vi "Servo SSC.vi"(0 "VISA resource name":refnum<visa-resource-name>="COM1", 6 "Read":bool) -> ()   [LabVIEW 2011]
doc: "The Basic Serial Read and Write example performs a Serial Port Read, a Serial Port Write, or a combination of these actions. The user selects the actions (read or write) on the front panel. If both are selected, the VI will write the data first, read data, and then close the VISA session that is opened to the port. This VI will wait until the specified number of bytes is received at the port. Only the number of bytes specified will be read.\n\nINSTRUCTIONS:\n1) Select the serial resource and configuration parameters (baud rate, data bits, parity, stop bits, flow control).\n2) Select the operations to be performed. \n3) Connect the serial port to your device. If no device is available, perform a loopback test by doing one of the following. Short pins 2 and 3 on a RS-232 cable or short pin 4 to pin 8 and pin 5 to pin 9 on a RS-485/422 cable. \n4) Run the VI to see the data read. (The \"read string\" will match the \"string to write\" if a loopback test was performed.)\n\nNote: The parameters set for the serial port must match the parameters of the connected instrument or device. In this example, the bytes to read parameter specifies the number of bytes that the serial port reads. If there were more bytes at the port than the number specified in bytes to read, those bytes would not be read. Also, if you specify to read more bytes than the number of bytes actually read, you might receive a timeout error message.\n\nOn the block diagram, the Configure Serial Port VI sets the configuration parameters. The front panel displays the controls used to configure the basic parameters, such as baud rate, data bits, and parity. Constants configure the other parameters the user probably does not need set. After the VISA Configure Serial Port VI opens the VISA session and configures the port, the VI passes the VISA resource name to other VIs that perform operations on that VISA resource. The VISA Write function sends a command to the serial device and the VISA Read function returns data based on the command. The VISA Close function then closes the reference to the serial device. It is important to close the reference; otherwise communication through with that port through protocols other than VISA might not be possible."
uses:
  <vilib>/Instr/_visa.llb/VISA Configure Serial Port (Instr).vi
panel:
  out "value 2":u8
  in  "delay before read (ms)":u32=25
  in  "string to write":string="va \n"
  out "bytes read":u32
  out "read string":string
  out "value 1":u8
  out "Waveform Chart":T1(graph)
  in  "SERVO 4":dbl(knob)=1500.0 scale=500.0..2500.0
  in  "SERVO 3":dbl(knob)=1500.0 scale=500.0..2500.0
  in  "SERVO 2":dbl(knob)=1500.0 scale=500.0..2500.0
  in  "SERVO 1":dbl(knob)=1500.0 scale=500.0..2500.0
  in  "SERVO 0":dbl(knob)=1500.0 scale=500.0..2500.0
  in  "Initial":bool
  in  "Time":dbl=500.0
  in  "Write":bool
  out "Result":string
  in  "stop":bool
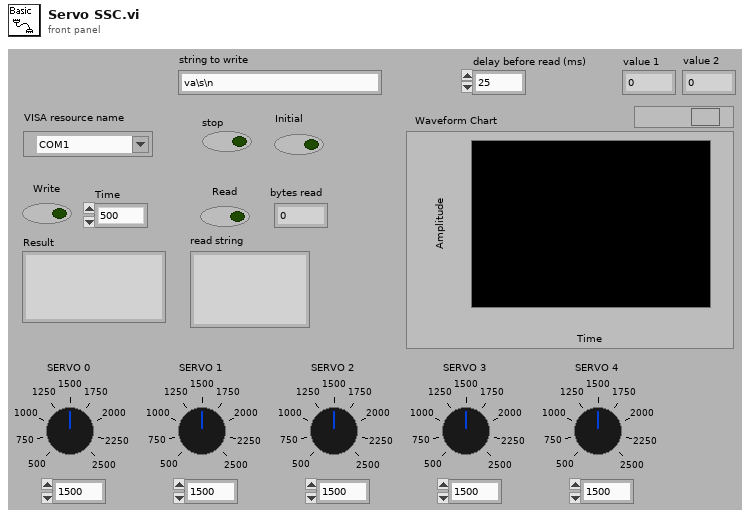
[diagram p1: front panel]
types:
  T1 = cluster{"unsigned byte array[0]":u8, "unsigned byte array[1]":u8, "unsigned byte array[2]":u8, "unsigned byte array[3]":u8, "unsigned byte array[4]":u8, "unsigned byte array[5]":u8, "unsigned byte array[6]":u8, "unsigned byte array[7]":u8, "unsigned byte array[8]":u8, "unsigned byte array[9]":u8, "unsigned byte array[10]":u8, "unsigned byte array[11]":u8, "unsigned byte array[12]":u8, "unsigned byte array[13]":u8, "unsigned byte array[14]":u8, "unsigned byte array[15]":u8, "unsigned byte array[16]":u8, "unsigned byte array[17]":u8}
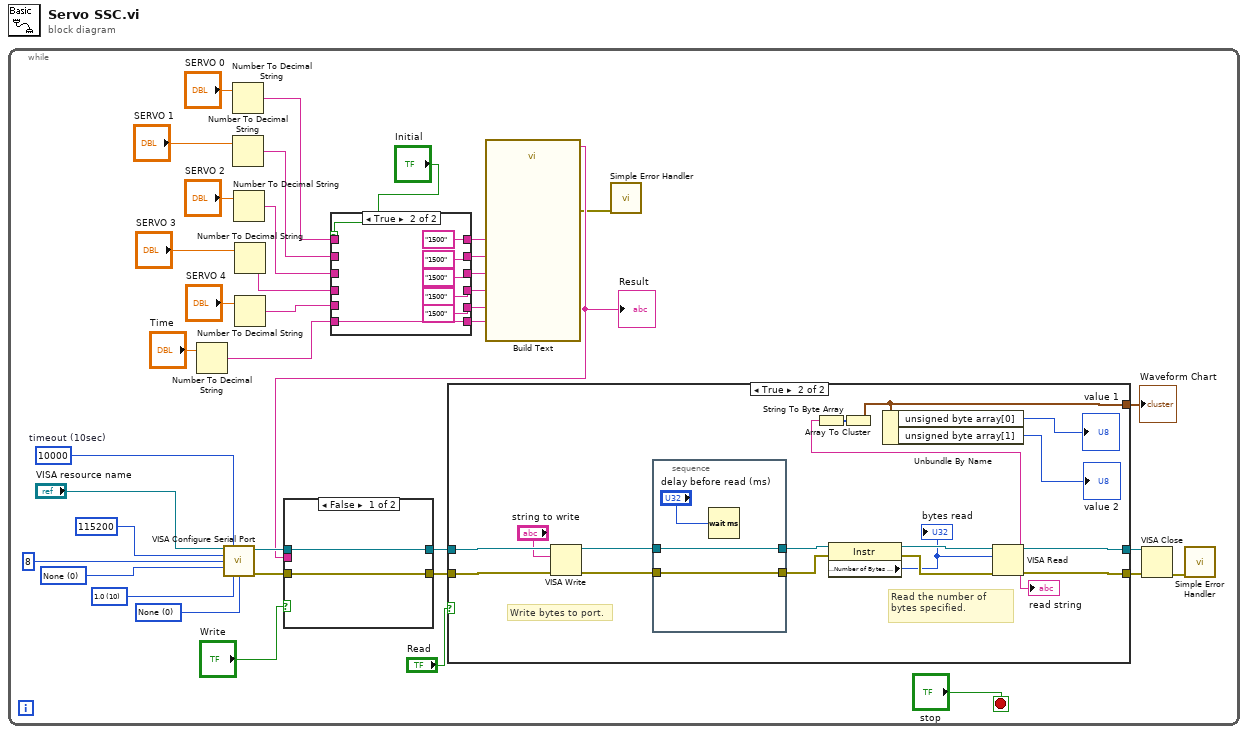
[diagram p0: block diagram]
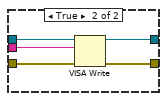
[diagram p3: hidden frame]
diagram:
  n1 = while {
    stop <- "stop" stop-if-true
    w33 = u16 0 items=["None"=0, "XON/XOFF"=1, "RTS/CTS"=2, "DTR/DSR"=4] ("flow control")
    w34 = u16 10 items=["1.0"=10, "1.5"=15, "2.0"=20] ("stop bits")
    w36 = u16 0 items=["None", "Odd", "Even", "Mark", "Space"] ("parity")
    w35 = u32 10000  # timeout (10sec)
    n2 = Number To Decimal String(number="Time") -> (decimal integer string=w21:string)  [unwired: 1 in]
    n3 = call-poly "VISA Configure Serial Port"("VISA resource name"="VISA resource name", "timeout (10sec)"=w35, "baud rate (9600)"=u32 115200 ("baud rate"), "data bits (8)"=u16 8 ("data bits"), "parity (0:none)"=w36, "stop bits (10: 1 bit)"=w34, "flow control (0:none)"=w33) -> ("VISA resource name out"=w31:refnum<visa-resource-name>, "error out"=w30:errorcluster)  [unwired: 7 in]
    n4 = Number To Decimal String(number="SERVO 0") -> (decimal integer string=w18:string)  [unwired: 1 in]
    n5 = Number To Decimal String(number="SERVO 1") -> (decimal integer string=w19:string)  [unwired: 1 in]
    n6 = Number To Decimal String(number="SERVO 2") -> (decimal integer string=w20:string)  [unwired: 1 in]
    n7 = Number To Decimal String(number="SERVO 3") -> (decimal integer string=w23:string)  [unwired: 1 in]
    n8 = Number To Decimal String(number="SERVO 4") -> (decimal integer string=w22:string)  [unwired: 1 in]
    n9 = case shown="True" "Initial" {
      tunnel: w23 -> [w43 _]
      tunnel: w22 -> [w44 _]
      tunnel: w21 -> [w45 w51]
      tunnel: w20 -> [w42 _]
      tunnel: w19 -> [w41 _]
      tunnel: w18 -> [w40 _]
      tunnel: [w45 w51] -> w17
      tunnel: [w44 "1500"] -> w16
      tunnel: [w43 "1500"] -> w15
      tunnel: [w42 "1500"] -> w14
      tunnel: [w41 "1500"] -> w13
      tunnel: [w40 "1500"] -> w12
      frame False {
      }
      frame True {
      }
    }
    n10 = call "Build Text"("pwm3"=w15, "time"=w17, "pwm0"=w12, "pwm1"=w13, "pwm2"=w14, "pwm4"=w16) -> ("Result"=w25:string, "error out"=w11:errorcluster)  [unwired: 8 in]
    "Result" <- w25
    n11 = case shown="False" "Write" {
      tunnel: w31 -> [w53 w58]
      tunnel: w30 -> [w52 w57]
      tunnel: [w53 w56] -> w29
      tunnel: [w52 w55] -> w28
      tunnel: w25 -> [_ w54]
      frame False {
      }
      frame True {
        n12 = VISA Write(VISA resource name=w58, write buffer=w54, error in (no error)=w57) -> (VISA resource name out=w56:refnum<visa-resource-name>, error out=w55:errorcluster)  [unwired: 1 out]
      }
    }
    n13 = case shown="True" "Read" {
      tunnel: w28 -> [w60 w72]
      tunnel: [w60 w66] -> w3
      tunnel: [w59 w67] -> w4
      tunnel: w29 -> [w59 w73]
      tunnel: [_ w69] -> w1
      frame False {
      }
      frame True {
        # "Read the number of bytes specified."
        # "Write bytes to port."
        n14 = VISA Write(VISA resource name=w73, write buffer="string to write", error in (no error)=w72) -> (VISA resource name out=w75:refnum<visa-resource-name>, error out=w77:errorcluster)  [unwired: 1 out]
        n15 = stacked-sequence {
          tunnel: w77 -> [w80]
          tunnel: [w80] -> w76
          tunnel: w75 -> [w79]
          tunnel: [w79] -> w74
          frame #0 {
            n16 = Wait (ms)(milliseconds to wait="delay before read (ms)") -> ()  [unwired: 1 out]
          }
        }
        n17 = property class="Instr"(reference=w74, error in=w76) -> (reference out=w64:refnum<visa-resource-name>, error out=w63:errorcluster, "Serial Settings:Number of Bytes at Serial Port"=w62:u32)
        "bytes read" <- w62
        n18 = VISA Read(VISA resource name=w64, byte count=w62, error in (no error)=w63) -> (VISA resource name out=w67:refnum<visa-resource-name>, read buffer=w70:string, error out=w66:errorcluster)  [unwired: 1 out]
        "read string" <- w70
        n19 = String To Byte Array(string=w70) -> (unsigned byte array=w71:u8[])
        n20 = Array To Cluster(array=w71) -> (cluster=w69:T1)
        n21 = Unbundle By Name(w69) -> ("unsigned byte array[0]"=→"value 1":u8, "unsigned byte array[1]"=→"value 2":u8)
      }
    }
    "Waveform Chart" <- w1
    n22 = call <vilib>:"Simple Error Handler.vi"("error in (no error)"=w11) -> ()  [unwired: 4 in, 5 out]
    n23 = VISA Close(VISA resource name=w4, error in (no error)=w3) -> (error out=w37:errorcluster)
    n24 = call <vilib>:"Simple Error Handler.vi"("error in (no error)"=w37) -> ()  [unwired: 4 in, 5 out]
  }
